vi "beginTableWith2ndStikerPlay.vi"(8 "error in (no error)":errorcluster, 10 "Game":refnum<class "Game.lvclass">, 11 "TableWith2ndStrikerPlay in":refnum<class "TableWith2ndStrikerPlay.lvclass">) -> (0 "error out":errorcluster, 2 "BeginTableWith2ndStriker?":bool, 3 "TableWith2ndStrikerPlay out":refnum<class "TableWith2ndStrikerPlay.lvclass">)   [LabVIEW 2023, in "TableWith2ndStrikerPlay.lvclass"]
uses:
  TableWith2ndStrikerPlay.lvclass
  Game_class/Game.lvclass
  Referee_class/command_interpreted.ctl
  Team_class/OffensivePlay.ctl
  Game_class/Game.lvclass/Game.ctl
  Referee_class/Referee.lvclass/Referee.ctl
  Object_class/Object.lvclass/Object.ctl
  Parameters_class/Parameters.lvclass/Parameters.ctl
  Team_class/Team.lvclass/Team.ctl
  Game_class/Read Referee.vi
  Game_class/Read Utilities.lvclass.vi
  Game_class/Read BallRef.vi
  Game_class/Read Parameters.lvclass.vi
  Game_class/Read FieldRef.vi
  Game_class/Read OffensiveTeam.vi
  Team_class/Read RobotRef.vi
  Parameters_class/Read AttakingOurselves.vi
  Object_class/Read x.vi
  Object_class/Read y.vi
  Referee_class/Read command_interpreted.vi
  Team_class/Read OffensivePlay.vi
  Ally_class/Ally.lvclass
  Ball_class/Ball.lvclass
  Robot_class/Robot.lvclass
  Referee_class/Referee.lvclass
  Utilities_class/Utilities.lvclass
  Parameters_class/Parameters.lvclass
  Field_class/Field.lvclass
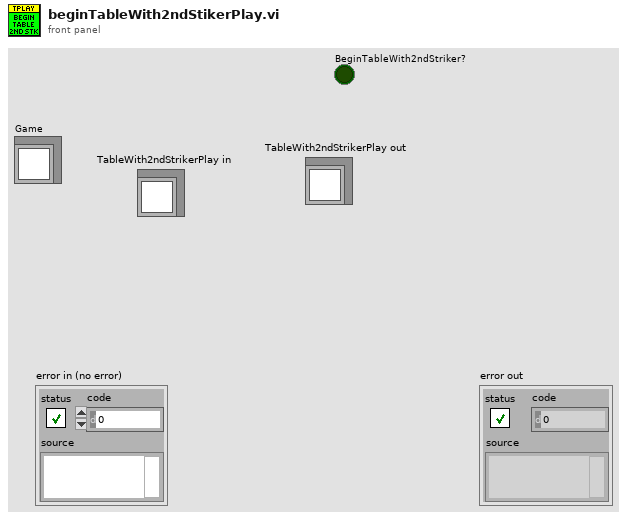
[diagram p1: front panel]
types:
  T1 = typedef "OffensivePlay.ctl" = enum16{"TableWithStriker", "TableWith2ndStrikerPlay", "PrepareDoublePass", "PrepareRollToPass", "SimplePass", "PreparePass", "PassToStriker", "BallOutOfField", "PassTo2ndStriker", "StopOffensive", "Prepare Penalty Enemy", "EnemyPossessionAtEnemyField", "EnemyPossesionAtOurField", "TestPlay", "PreparePenaltyAlly", "KickPenaltyAlly", "PrepareKickoffAlly", "PrepareKickoffEnemy", "IndirectEnemy", "DirectEnemy", "NormalGame", "DirectKick", "Pass", "Halt", "Timeout", "PassPlay", "PenaltyEnemy"}
  T2 = typedef "command_interpreted.ctl" = enum16{"Goal Ally", "Goal Enemy", "Ball Placement Enemy", "Ball Placement Ally", "Normal Half Time", "Extra Time  Break", "Extra Half Time", "None", "Post Game", "PKA Normal Start", "Prepare Kickoff Ally", "PKE Normal Start", "Prepare Kickoff Enemy", "Force Start", "Halt", "Timeout", "Prepare Penalty Ally", "Prepare Penalty Enemy", "PPA NormalStart", "PPE Normal Start", "Indirect Free Ally", "Direct Free Enemy", "Direct Free Ally", "Indirect Free Enemy", "Stop"}
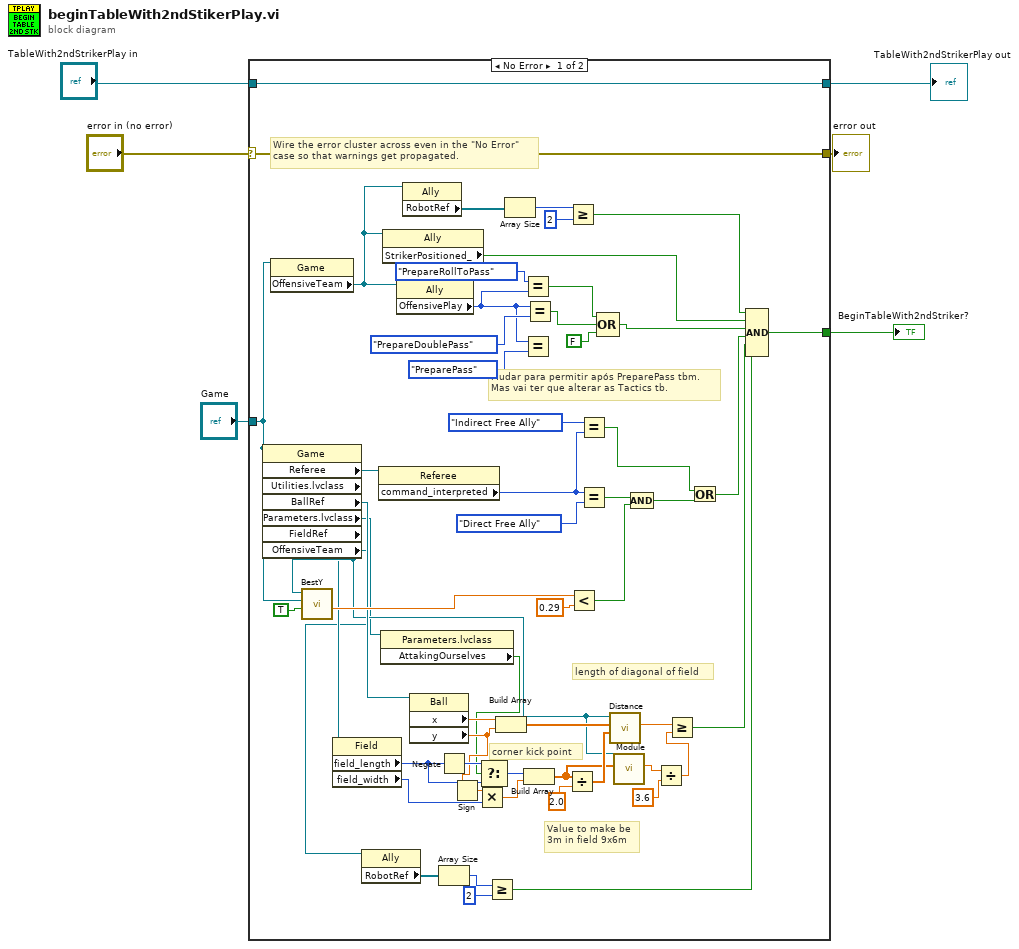
[diagram p0: block diagram]
diagram:
  n1 = case shown="No Error" "error in (no error)" {
    selector: "error in (no error)" -> [w62 w65]
    tunnel: [w62 w65] -> w5
    tunnel: [w63 w64] -> w1
    tunnel: "TableWith2ndStrikerPlay in" -> [w63 w64]
    tunnel: "Game" -> [w53 _]
    tunnel: [w52 _] -> w3
    frame No Error {
      # "Mudar para permitir após PreparePass tbm.\nMas vai ter que alterar as Tactics tb."
      # "corner kick point"
      # "length of diagonal of field"
      # "Value to make be\n3m in field 9x6m"
      # "Wire the error cluster across even in the \"No Error\"\ncase so that warnings get propagated."
      n2 = property class="Game"(reference=w53) -> ("Referee"=w61:refnum<class "Referee.lvclass">, "Utilities.lvclass"=w18:refnum<class "Utilities.lvclass">, "BallRef"=w20:refnum<class "Ball.lvclass">, "Parameters.lvclass"=w17:refnum<class "Parameters.lvclass">, "FieldRef"=w15:refnum<class "Field.lvclass">, "OffensiveTeam"=w14:refnum<class "Ally.lvclass">)  [unwired: 1 in, 2 out]
      n3 = property class="Game"(reference=w53) -> ("OffensiveTeam"=w42:refnum<class "Ally.lvclass">)  [unwired: 1 in, 2 out]
      n4 = call "BestY.vi"("Utilities in"=w18, "Game"=w53, "inimigos"=TRUE) -> ("Gap kick"=w55:dbl)  [unwired: 2 in, 4 out]
      n5 = property class="Field"(reference=w15) -> ("field_length"=w32:i32, "field_width"=w31:i32)  [unwired: 1 in, 2 out]
      n6 = property class="Ally"(reference=w14) -> ("RobotRef"=w13:refnum<class "Robot.lvclass">[])  [unwired: 1 in, 2 out]
      n7 = property class="Referee"(reference=w61) -> ("command_interpreted"=w59:T2)  [unwired: 1 in, 2 out]
      n8 = property class="Parameters.lvclass"(reference=w17) -> ("AttakingOurselves"=w16:bool)  [unwired: 1 in, 2 out]
      n9 = property class="Ally"(reference=w42) -> ("StrikerPositioned_"=w51:bool)  [unwired: 1 in, 2 out]
      n10 = property class="Ally"(reference=w42) -> ("OffensivePlay"=w9:T1)  [unwired: 1 in, 2 out]
      n11 = property class="Ally"(reference=w42) -> ("RobotRef"=w41:refnum<class "Robot.lvclass">[])  [unwired: 1 in, 2 out]
      n12 = property class="Ball"(reference=w20) -> ("x"=w36:dbl, "y"=w30:dbl)  [unwired: 1 in, 2 out]
      n13 = Negate(x=w32) -> (-x=w34:i32)
      n14 = Array Size(array=w13) -> (size(s)=w12:i32)
      n15 = Sign(1:w30) -> (0:w29:dbl)
      n16 = Multiply(x=w29, y=w31) -> (x*y=w28:dbl)
      n17 = Select(t=w34, s=w16, f=w32) -> (s? t:f=w33:i32)
      n18 = Greater Or Equal?(x=w12, y=2) -> (x >= y?=w10:bool)
      n19 = Build Array(w36, w30) -> (w35:dbl[])
      n20 = Array Size(array=w41) -> (size(s)=w40:i32)
      n21 = Equal?(x=OffensivePlay."PrepareRollToPass" ("OffensivePlay"), y=w9) -> (x = y?=w44:bool)
      n22 = Equal?(x=w9, y=OffensivePlay."PreparePass" ("OffensivePlay")) -> ()  [unwired: 1 out]
      n23 = Build Array(w33, w28) -> (w24:dbl[])
      n24 = Equal?(x=w9, y=OffensivePlay."PrepareDoublePass" ("OffensivePlay")) -> (x = y?=w45:bool)
      n25 = Divide(x=w24, y=2.0) -> (x/y=w25:dbl[])
      n26 = Greater Or Equal?(x=w40, y=2) -> (x >= y?=w38:bool)
      n27 = Less?(x=w55, y=0.29 ("Gap kick")) -> (x < y?=w54:bool)
      n28 = Equal?(x=command_interpreted."Indirect Free Ally" ("command_interpreted"), y=w59) -> (x = y?=w48:bool)
      n29 = Equal?(x=w59, y=command_interpreted."Direct Free Ally" ("command_interpreted")) -> (x = y?=w50:bool)
      n30 = Compound Arithmetic op=OR(w44, w45, FALSE) -> (w43:bool)
      n31 = call-dynamic "Distance.vi"("P1"=w25, "P2"=w35, "Utilities in"=w18) -> ("Distance"=w26:dbl)  [unwired: 6 in, 2 out]
      n32 = call-dynamic "Module.vi"("2D vector"=w24, "Utilities in"=w18) -> ("Modulo"=w23:dbl)  [unwired: 7 in, 2 out]
      n33 = Compound Arithmetic op=AND(w50, w54) -> (w49:bool)
      n34 = Divide(x=w23, y=3.6) -> (x/y=w21:dbl)
      n35 = Greater Or Equal?(x=w26, y=w21) -> (x >= y?=w19:bool)
      n36 = Or(x=w48, y=w49) -> (x .or. y?=w37:bool)
      n37 = Compound Arithmetic op=AND(w38, w51, w43, w37, w19, w10) -> (w52:bool)
    }
    frame Error {
    }
  }
  "error out" <- w5
  "BeginTableWith2ndStriker?" <- w3
  "TableWith2ndStrikerPlay out" <- w1
